vi "List to Array.vi"(4 "error in (no error)":errorcluster, 5 "List":string, 7 "Separator (,)":string=",") -> (0 "error out":errorcluster, 1 "Output Number Array":dbl[](array[numeric]) format="%.2f", 3 "Output String Array":string[](array[string]))   [LabVIEW 2013]
doc: "Given a List of strings separated by a Separator, this VI returns the List as a String Array. If the strings are numbers, a Number Array is also returned."
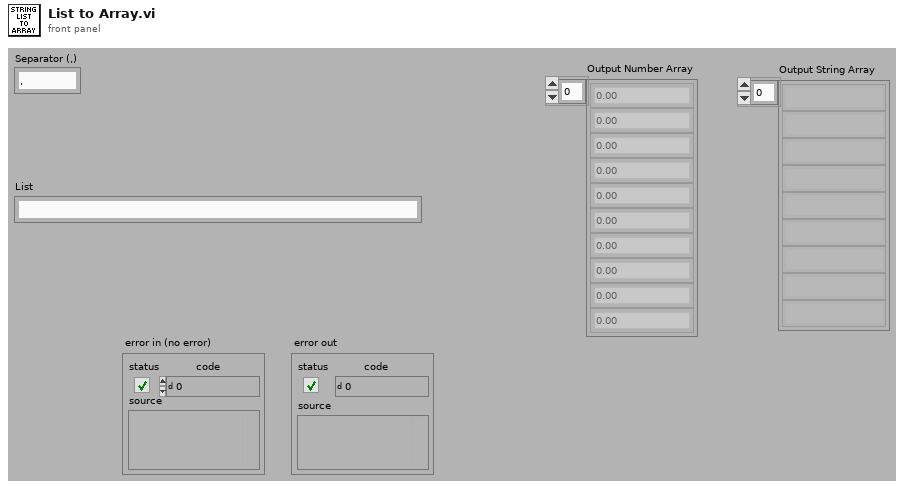
[diagram p1: front panel]
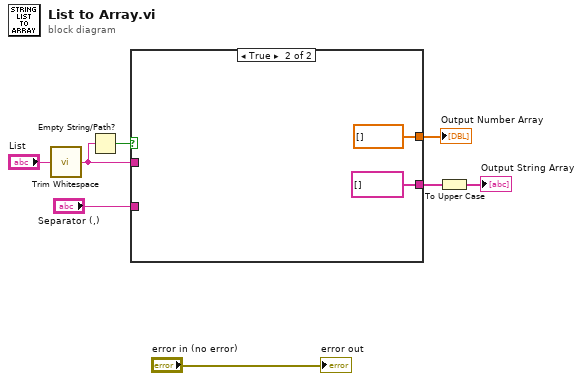
[diagram p0: block diagram]
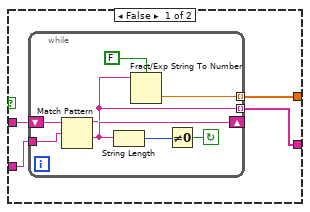
[diagram p2: hidden frame]
diagram:
  n1 = call <vilib>:"Trim Whitespace.vi"("string"="List") -> ("trimmed string"=w5:string)  [unwired: 1 in]
  n2 = Empty String/Path?(string/path=w5) -> (empty?=w4:bool)
  n3 = case shown="True" w4 {
    tunnel: "Separator (,)" -> [w12 _]
    tunnel: [w11 string[] []] -> w3
    tunnel: [w10 dbl[] []] -> w7
    tunnel: w5 -> [w9 _]
    frame False {
      n4 = while {
        tunnel: w12 -> [w14]
        tunnel: [w15] -> w11 mode=indexing
        tunnel: [w17] -> w10 mode=indexing
        shift-left: w9 -> [w18]
        shift-right: [w16] -> _
        stop <- w20 continue-if-true
        n5 = Match Pattern(string=w18, regular expression=w14) -> (before substring=w15:string, after substring=w16:string)  [unwired: 1 in, 2 out]
        n6 = String Length(string=w16) -> (length=w19:i32)
        n7 = Fract/Exp String To Number(use system decimal point (T)=FALSE, string=w15) -> (number=w17:dbl)  [unwired: 2 in, 1 out]
        n8 = Not Equal To 0?(x=w19) -> (x != 0?=w20:bool)
      }
    }
    frame True {
    }
  }
  "Output Number Array" <- w7
  n9 = To Upper Case(1:w3) -> (0:→"Output String Array":string[])
  "error out" <- "error in (no error)"
